vi "Extract time from string.vi"(0 "ics time string":string, 11 "Error In":errorcluster) -> (4 "Time and Date":timestamp, 15 "Error Out":errorcluster)   [LabVIEW 2016]
doc: "Extract time from string VI extracts time from ics format string."
uses:
  <vilib>/Utility/miscctls.llb/LVDateTimeRec.ctl
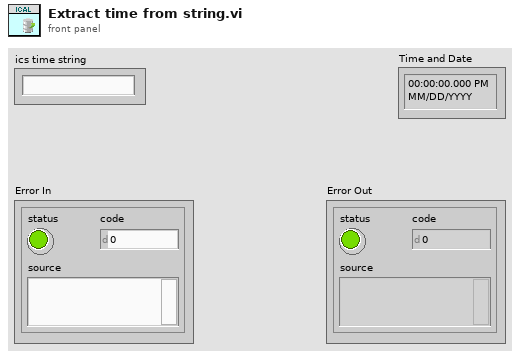
[diagram p1: front panel]
types:
  T1 = typedef "LVDateTimeRec.ctl" = cluster{"fractional second":dbl, "second":i32, "minute":i32, "hour":i32, "day of month":i32, "month":i32, "year":i32, "day of week":i32, "day of year":i32, "DST":i32}
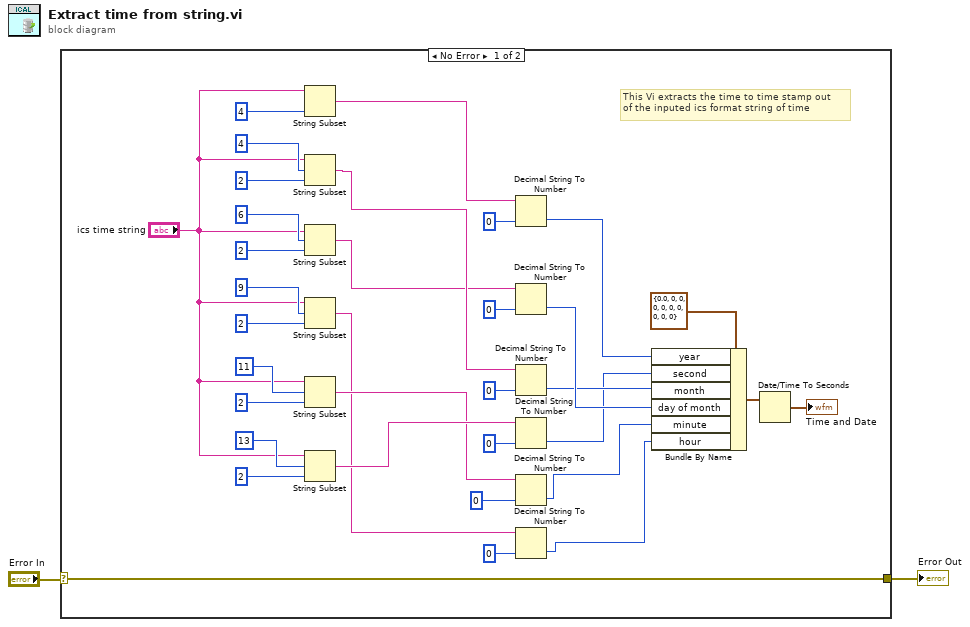
[diagram p0: block diagram]
diagram:
  n1 = case shown="No Error" "Error In" {
    selector: "Error In" -> [w4 w37]
    tunnel: [w4 w37] -> w1
    frame No Error {
      # "This Vi extracts the time to time stamp out \nof the inputed ics format string of time"
      n2 = String Subset(string="ics time string", length (rest)=4 ("length (rest)")) -> (substring=w11:string)  [unwired: 1 in]
      n3 = String Subset(string="ics time string", offset (0)=4, length (rest)=2 ("length (rest)")) -> (substring=w10:string)
      n4 = String Subset(string="ics time string", offset (0)=6, length (rest)=2 ("length (rest)")) -> (substring=w9:string)
      n5 = String Subset(string="ics time string", offset (0)=9, length (rest)=2 ("length (rest)")) -> (substring=w12:string)
      n6 = String Subset(string="ics time string", offset (0)=11, length (rest)=2 ("length (rest)")) -> (substring=w14:string)
      n7 = String Subset(string="ics time string", offset (0)=13, length (rest)=2 ("length (rest)")) -> (substring=w31:string)
      n8 = Decimal String To Number(string=w11, default (0L)=0 ("Hours")) -> (number=w35:i32)  [unwired: 1 in, 1 out]
      n9 = Decimal String To Number(string=w9, default (0L)=0 ("Hours")) -> (number=w33:i32)  [unwired: 1 in, 1 out]
      n10 = Decimal String To Number(string=w10, default (0L)=0 ("Hours")) -> (number=w32:i32)  [unwired: 1 in, 1 out]
      n11 = Decimal String To Number(string=w31, default (0L)=0 ("Hours")) -> (number=w8:i32)  [unwired: 1 in, 1 out]
      n12 = Decimal String To Number(string=w14, default (0L)=0 ("Hours")) -> (number=w6:i32)  [unwired: 1 in, 1 out]
      n13 = Decimal String To Number(string=w12, default (0L)=0 ("Hours")) -> (number=w5:i32)  [unwired: 1 in, 1 out]
      n14 = Bundle By Name(cluster=T1 {"fractional second"=0.0, "second"=0, "minute"=0, "hour"=0, "day of month"=0, "month"=0, "year"=0, "day of week"=0, "day of year"=0, "DST"=0} ("date time rec"), "year"=w35, "second"=w8, "month"=w32, "day of month"=w33, "minute"=w6, "hour"=w5) -> (w36:T1)
      n15 = Date/Time To Seconds(2:w36) -> (0:→"Time and Date":timestamp)  [unwired: 1 in]
    }
    frame Error {
    }
  }
  "Error Out" <- w1
